vi "Turn Off All Outputs.vi"(8 "error in (no error)":errorcluster, 11 "NI-DAQ in":refnum<class "NI-DAQ.lvclass">) -> (0 "error out":errorcluster, 3 "NI-DAQ out":refnum<class "NI-DAQ.lvclass">)   [LabVIEW 2020, in "NI-DAQ.lvclass"]
uses:
  NI-DAQ.lvclass
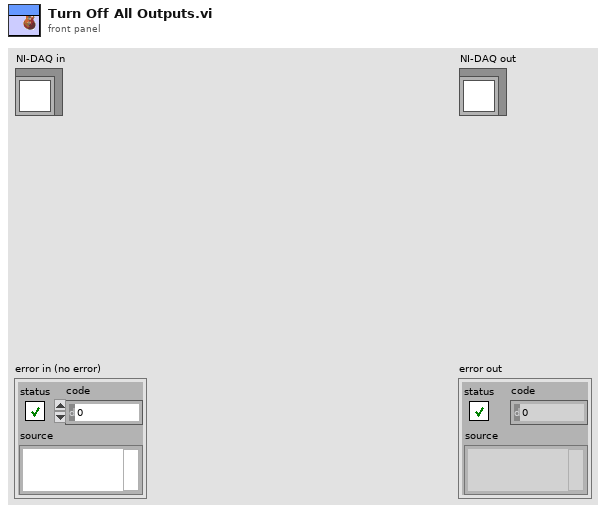
[diagram p1: front panel]
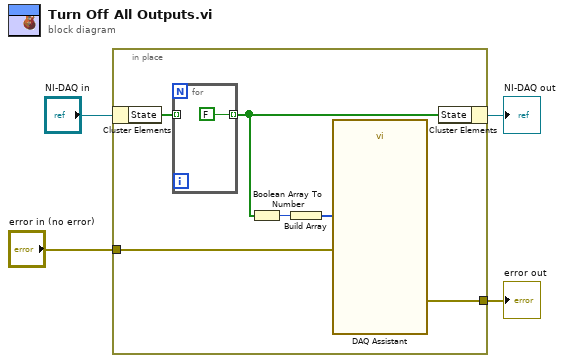
[diagram p0: block diagram]
diagram:
  n1 = in-place {
    in-place-border: [w6] -> w2
    in-place-border: "error in (no error)" -> [w5]
    n2 = in-place-cluster #1("NI-DAQ in") -> ("State"=w10:bool[])
    n3 = for {
      tunnel: w10 -> [_] mode=indexing
      tunnel: [FALSE] -> w7 mode=indexing
    }
    n4 = Boolean Array To Number(Boolean array=w7) -> (number=w9:u32)
    n5 = Build Array(w9) -> (w8:u32[])
    n6 = call "DAQ Assistant"("data"=w8, "error in"=w5) -> ("error out"=w6:errorcluster)  [unwired: 16 in, 1 out]
    n7 = in-place-cluster #1("State"=w7) -> (→"NI-DAQ out":refnum<class "NI-DAQ.lvclass">)
  }
  "error out" <- w2
